vi "Ist mit Soll vergleichen Alarme.vi"(8 "error in (no error)":errorcluster caption="Fehler (Eingang, kein Fehler)", 11 "Schneider Steuerung PNS Eingang":refnum<class "Schneider Steuerung PNS.lvclass">) -> (0 "error out":errorcluster caption="Fehler (Ausgang)", 2 "Werte":cluster{u16[], u16[]}, 3 "Schneider Steuerung PNS Ausgang":refnum<class "Schneider Steuerung PNS.lvclass">)   [LabVIEW 2020, in "Schneider Steuerung PNS.lvclass"]
uses:
  Schneider Steuerung PNS.lvclass
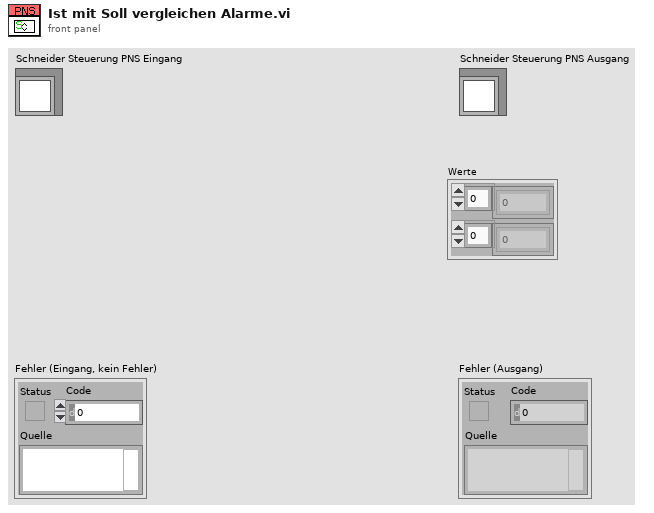
[diagram p1: front panel]
types:
  T1 = typedef "Steuerung PNS.lvclass/Anlegengrenzwerte PNS.ctl" = cluster{"Filter:":T2, "Ventilplatte:":T2, "Heizleitung 1:":T2, "Heizleitung 2:":T2, "Heizleitung 3:":T2, "Heizleitung 4:":T2, "Heizleitung 5:":T2, "Heizleitung 6:":T2}
  T2 = typedef "Steuerung PNS.lvclass/Anlagengrenzwerte Parameteranzeige.ctl" = cluster{"Sollwert":T3, "Warn-Min":T3, "Warn-Max":T3, "Abschalt-Min":T3, "Abschalt-Max":T3, "Regler":u16, "AnlagenParameter":string}
  T3 = typedef "Zahlen-Eingabefeld.ctl" = sgl
  T4 = typedef "Steuerung PNS.lvclass/Alarme.ctl" = cluster{"Alarm Filter max":u16, "Alarm Filter min":u16, "Alarm Ventilplatte max":u16, "Alarm Ventilplatte min":u16, "Alarm HL1 max":u16, "Alarm HL1 min":u16, "Alarm HL2 max":u16, "Alarm HL2 min":u16, "Alarm HL3 max":u16, "Alarm HL3 min":u16, "Alarm HL4 max":u16, "Alarm HL4 min":u16, "Alarm HL5 max":u16, "Alarm HL5 min":u16, "Alarm HL6 max":u16, "Alarm HL6 min":u16}
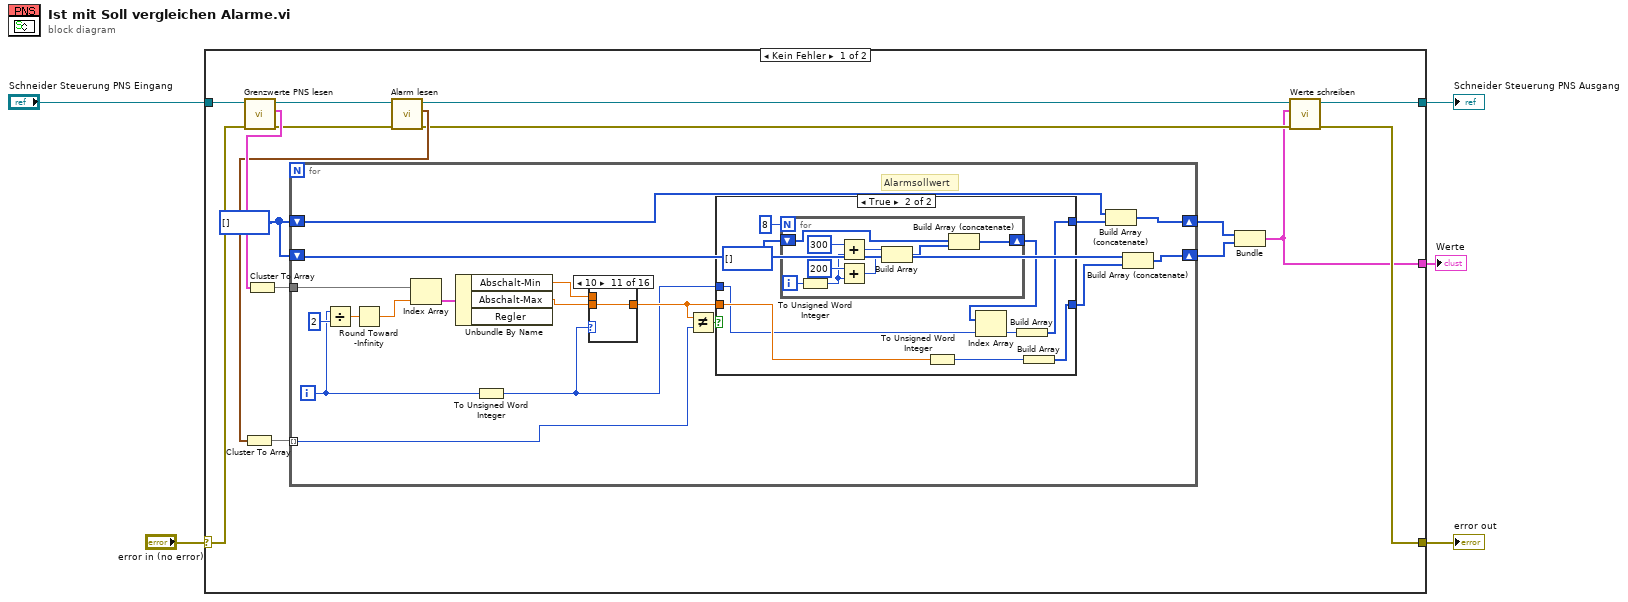
[diagram p0: block diagram]
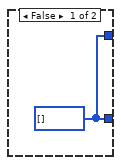
[diagram p2: hidden frame]
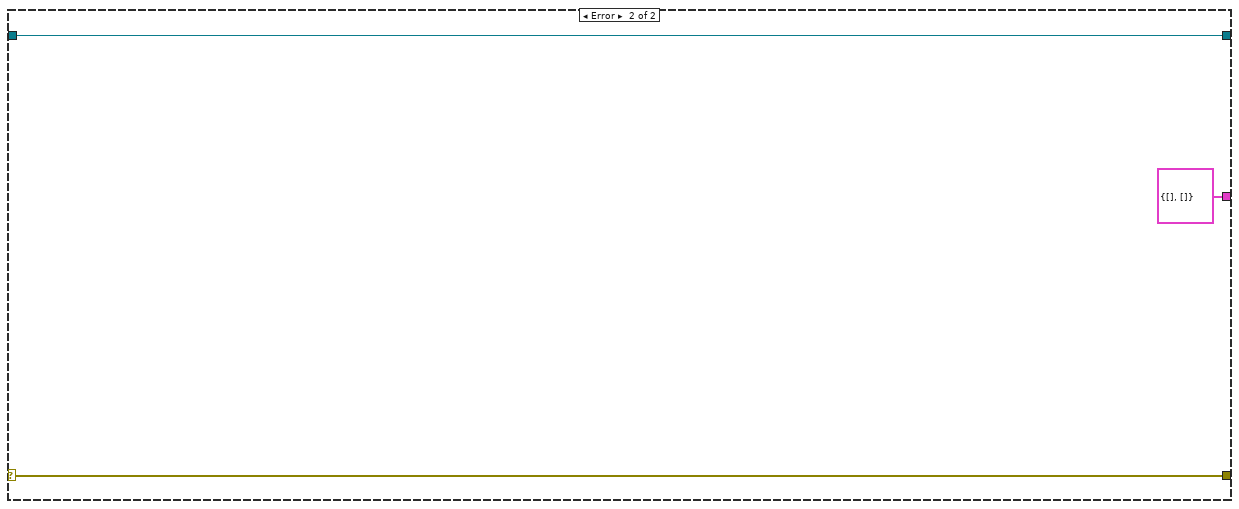
[diagram p18: hidden frame]
diagram:
  n1 = case shown="Kein Fehler" "error in (no error)" {
    selector: "error in (no error)" -> [w8 w77]
    tunnel: [w7 w77] -> w4
    tunnel: [w10 w76] -> w2
    tunnel: "Schneider Steuerung PNS Eingang" -> [w21 w76]
    tunnel: [w6 cluster{u16[], u16[]} {[], []}] -> w1
    frame No Error {
      w19 = u16[] []
      n2 = call-dynamic "Grenzwerte PNS lesen.vi"("error in (no error)"=w8, "Steuerung PNS (Eingang)"=w21) -> ("error out"=w15:errorcluster, "Grenzwerte PNS"=w17:T1, "Steuerung PNS (Ausgang)"=w18:refnum<class "Schneider Steuerung PNS.lvclass">)  [unwired: 7 in]
      n3 = Cluster To Array(cluster=w17) -> (array=w20:T2[])
      n4 = call-dynamic "Alarm lesen.vi"("error in (no error)"=w15, "Steuerung PNS (Eingang)"=w18) -> ("error out"=w9:errorcluster, "Alarm"=w14:T4, "Steuerung PNS (Ausgang)"=w16:refnum<class "Schneider Steuerung PNS.lvclass">)  [unwired: 7 in]
      n5 = Cluster To Array(cluster=w14) -> (array=w13:u16[])
      n6 = for {
        tunnel: w20 -> [w39]
        tunnel: w13 -> [w22] mode=indexing
        shift-right: [w25] -> w12
        shift-left: w19 -> [w31]
        shift-right: [w29] -> w11
        shift-left: w19 -> [w28]
        i -> [w23]
        # "Alarmsollwert"
        n7 = Divide(x=w23, y=2) -> (x/y=w36:dbl)
        n8 = Round Toward -Infinity(1:w36) -> (0:w35:dbl)
        n9 = Index Array(array=w39, index=w35) -> (element=w38:T2)
        n10 = Unbundle By Name(w38) -> ("Abschalt-Min"=w34:T3, "Abschalt-Max"=w33:T3)  [unwired: 1 out]
        n11 = To Unsigned Word Integer(number=w23) -> (unsigned 16bit integer=w24:u16)
        n12 = case shown="10" w24 {
          tunnel: w34 -> [_ w60 _ w62 _ w64 _ w66 _ w68 _ w70 _ w72 _ w74]
          tunnel: w33 -> [w59 _ w61 _ w63 _ w65 _ w67 _ w69 _ w71 _ w73 _]
          tunnel: [w59 w60 w61 w62 w63 w64 w65 w66 w67 w68 w69 w70 w71 w72 w73 w74] -> w26
          frame 0, Default {
          }
          frame 1 {
          }
          frame 2 {
          }
          frame 3 {
          }
          frame 4 {
          }
          frame 5 {
          }
          frame 6 {
          }
          frame 7 {
          }
          frame 8 {
          }
          frame 9 {
          }
          frame 10 {
          }
          frame 11 {
          }
          frame 12 {
          }
          frame 13 {
          }
          frame 14 {
          }
          frame 15 {
          }
        }
        n13 = Not Equal?(x=w26, y=w22) -> (x != y?=w32:bool)
        n14 = case shown="True" w32 {
          tunnel: w26 -> [_ w49]
          tunnel: [w40 w43] -> w30
          tunnel: [w40 w47] -> w27
          tunnel: w24 -> [_ w42]
          frame False {
            w40 = u16[] []
          }
          frame True {
            n15 = for {
              N: 8 -> [_]
              shift-right: [w51] -> w45
              shift-left: u16[] [] -> [w54]
              i -> [w53]
              n16 = To Unsigned Word Integer(number=w53) -> (unsigned 16bit integer=w50:u16)
              n17 = Add(x=u16 300, y=w50) -> (x+y=w56:u16)
              n18 = Add(x=u16 200, y=w50) -> (x+y=w55:u16)
              n19 = Build Array(w56, w55) -> (w52:u16[])
              n20 = Build Array (concatenate)(w54, w52) -> (w51:u16[])
            }
            n21 = To Unsigned Word Integer(number=w49) -> (unsigned 16bit integer=w48:u16)
            n22 = Index Array(array=w45, index=w42) -> (element=w44:u16)
            n23 = Build Array(w44) -> (w43:u16[])
            n24 = Build Array(w48) -> (w47:u16[])
          }
        }
        n25 = Build Array (concatenate)(w31, w30) -> (w25:u16[])
        n26 = Build Array (concatenate)(w28, w27) -> (w29:u16[])
      }
      n27 = Bundle(w12, w11) -> (w6:cluster{u16[], u16[]})  [unwired: 1 in]
      n28 = call-dynamic "Werte schreiben.vi"("error in (no error)"=w9, "Werte"=w6, "Steuerung PNS (Eingang)"=w16) -> ("error out"=w7:errorcluster, "Steuerung PNS (Ausgang)"=w10:refnum<class "Schneider Steuerung PNS.lvclass">)  [unwired: 7 in]
    }
    frame Error {
    }
  }
  "error out" <- w4
  "Schneider Steuerung PNS Ausgang" <- w2
  "Werte" <- w1
